vi "JSON to LVObject - Error Input - Returns LabVIEW Object.vi"() -> ()   [LabVIEW 2017, in "Tests.lvlib"]
uses:
  Tests.lvlib
  Flatten To JSON Object/Flatten To JSON Object.lvclass
  Weather Forecast/Weather Forecast.lvclass
  <vilib>/Utility/error.llb/Error Cluster From Error Code.vi
  <vilib>/addons/_JKI Toolkits/Caraya/classes/Assert/Assert Equal Value and Type_Variant.vi
  <vilib>/ErrorRing/Error Ring.xnode
  <vilib>/addons/_JKI Toolkits/Caraya/classes/Test/Test.lvclass
  <vilib>/addons/_JKI Toolkits/Caraya/classes/Assert/Assert.lvclass
panel:
  out "error out":errorcluster
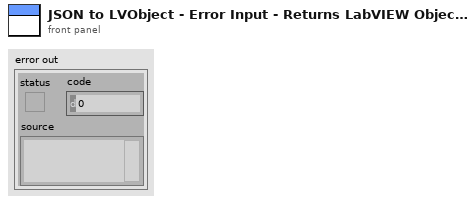
[diagram p1: front panel]
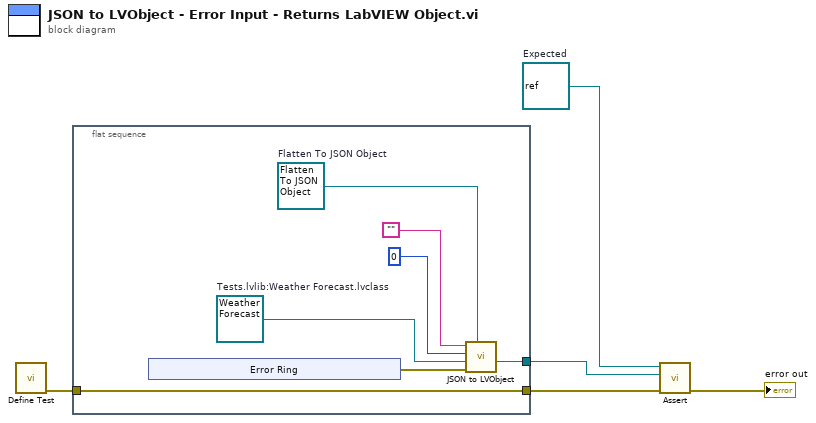
[diagram p0: block diagram]
diagram:
  w1 = refnum<class> refnum  # Expected
  n1 = call <vilib>:"Define Test.vi"() -> ("error out"=w4:errorcluster)  [unwired: 11 in]
  n2 = flat-sequence {
    tunnel: w4 -> [w10]
    tunnel: [w10] -> w3
    tunnel: [w8] -> w2
    frame #0 {
      w11 = refnum<class "Weather Forecast.lvclass"> refnum  # Tests.lvlib:Weather Forecast.lvclass
      w12 = refnum<class "Flatten To JSON Object.lvclass"> refnum  # Flatten To JSON Object
      n3 = xnode "Error Ring"() -> ("error out"=w9:errorcluster)
      n4 = call-dynamic "JSON to LVObject.vi"("Flatten To JSON Object in"=w12, "error in (no error)"=w9, "Object Type"=w11, "Offset"=0, "JSON"="") -> ("Object"=w8:refnum<class>)  [unwired: 5 in, 1 out]
    }
  }
  n5 = call-poly <vilib>:"Assert.vi"("error in (no error)"=w3, "Y"=w2, "X"=w1) -> ("error out"=→"error out":errorcluster)  [unwired: 8 in]
